vi "GoToControl.vi"(6 "Team":enum16{"Offensive", "Defensive", "Kepper"}(ring), 8 "error in (no error)":errorcluster, 9 "PID Gains Angle":T1={"proportional gain (Kc)"=5.0, "integral time (Ti, min)"=0.0, "derivative time (Td, min)"=-2.0}, 10 "PID Gains XY":T1={"proportional gain (Kc)"=0.005, "integral time (Ti, min)"=0.0, "derivative time (Td, min)"=-0.07}, 11 "Game in":refnum<class "Game.lvclass">) -> (0 "error out":errorcluster, 3 "Game out":refnum<class "Game.lvclass">)   [LabVIEW 2021, in "Game.lvclass"]
uses:
  Game.lvclass
  Game.lvclass/Game.ctl
  Team_class/Team.lvclass/Team.ctl
  Object_class/Object.lvclass/Object.ctl
  Robot_class/Robot.lvclass/Robot.ctl
  Object_class/Read x.vi
  Object_class/Read y.vi
  Robot_class/Read orientation.vi
  Robot_class/Read dest_x.vi
  Robot_class/Read dest_y.vi
  Robot_class/Read dest_orientation.vi
  Robot_class/Read id.vi
  Robot_class/Write v_tang.vi
  Robot_class/Write v_norm.vi
  Robot_class/Write v_ang.vi
  Write OffensiveTeam.vi
  Write DefensiveTeam.vi
  Write KeeperTeam.vi
  Team_class/Read RobotRef.vi
  Team_class/Write RobotRef.vi
  Ally_class/Ally.lvclass
  D:/RoboIme/horie/SSL_AI/Team_class/Team.lvclass
  Robot_class/Robot.lvclass
  D:/RoboIme/horie/SSL_AI/Object_class/Object.lvclass
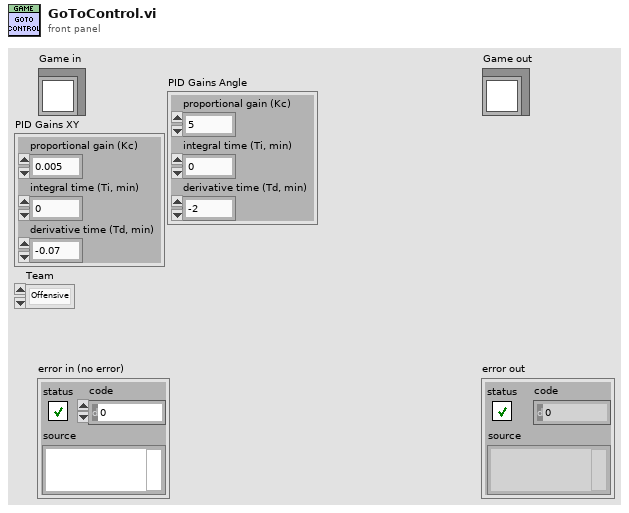
[diagram p1: front panel]
types:
  T1 = cluster{"proportional gain (Kc)":dbl, "integral time (Ti, min)":dbl, "derivative time (Td, min)":dbl}
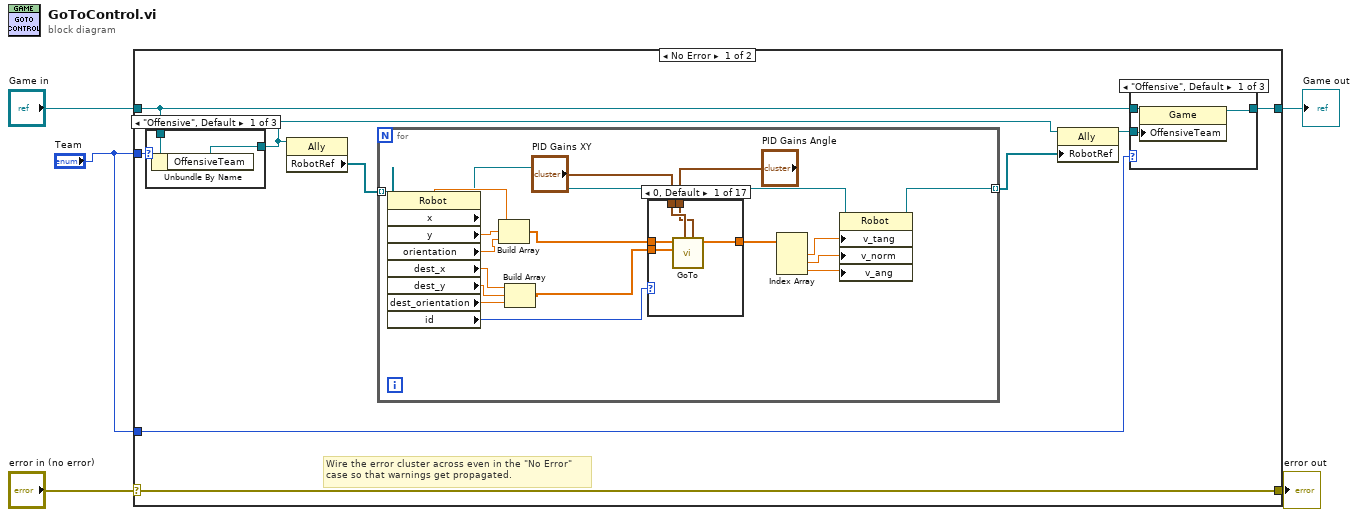
[diagram p0: block diagram]
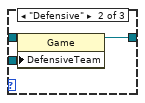
[diagram p2: hidden frame]
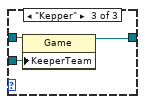
[diagram p3: hidden frame]
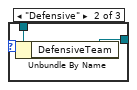
[diagram p4: hidden frame]
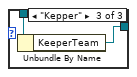
[diagram p5: hidden frame]
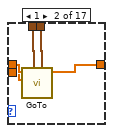
[diagram p6: hidden frame]
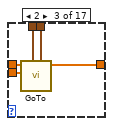
[diagram p7: hidden frame]
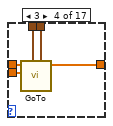
[diagram p8: hidden frame]
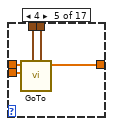
[diagram p9: hidden frame]
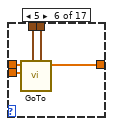
[diagram p10: hidden frame]
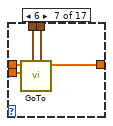
[diagram p11: hidden frame]
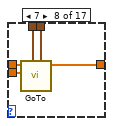
[diagram p12: hidden frame]
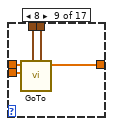
[diagram p13: hidden frame]
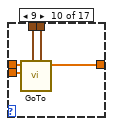
[diagram p14: hidden frame]
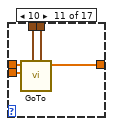
[diagram p15: hidden frame]
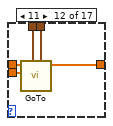
[diagram p16: hidden frame]
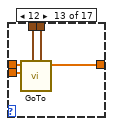
[diagram p17: hidden frame]
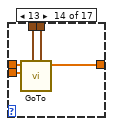
[diagram p18: hidden frame]
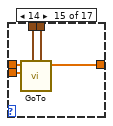
[diagram p19: hidden frame]
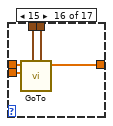
[diagram p20: hidden frame]
diagram:
  n1 = case shown="No Error" "error in (no error)" {
    selector: "error in (no error)" -> [w14 w134]
    tunnel: [w14 w134] -> w4
    tunnel: [w8 w133] -> w2
    tunnel: "Game in" -> [w10 w133]
    tunnel: "Team" -> [w7 _]
    tunnel: "Team" -> [w6 _]
    frame No Error {
      # "Wire the error cluster across even in the \"No Error\"\ncase so that warnings get propagated."
      n2 = case shown="\"Offensive\", Default" w7 {
        tunnel: [w24 w27 w28] -> w12
        tunnel: w10 -> [w25 w26 w29]
        frame "Offensive", Default {
          n3 = Unbundle By Name(w25) -> ("OffensiveTeam"=w24:refnum<class "Ally.lvclass">)
        }
        frame "Defensive" {
          n4 = Unbundle By Name(w26) -> ("DefensiveTeam"=w27:refnum<class "Ally.lvclass">)
        }
        frame "Kepper" {
          n5 = Unbundle By Name(w29) -> ("KeeperTeam"=w28:refnum<class "Ally.lvclass">)
        }
      }
      n6 = property class="Ally"(reference=w12) -> ("RobotRef"=w13:refnum<class "Robot.lvclass">[])  [unwired: 1 in, 2 out]
      n7 = for {
        tunnel: w13 -> [w47] mode=indexing
        tunnel: [w37] -> w11 mode=indexing
        n8 = property class="Robot"(reference=w47) -> (reference out=w42:refnum<class "Robot.lvclass">, "x"=w46:dbl, "y"=w45:dbl, "orientation"=w34:dbl, "dest_x"=w44:dbl, "dest_y"=w43:dbl, "dest_orientation"=w32:dbl, "id"=w30:i32)  [unwired: 1 in, 1 out]
        n9 = Build Array(w46, w45, w34) -> (w33:dbl[])
        n10 = Build Array(w44, w43, w32) -> (w31:dbl[])
        n11 = case shown="0, Default" w30 {
          tunnel: [w50 w57 w62 w67 w72 w77 w82 w87 w92 w97 w102 w107 w112 w117 w122 w127 w132] -> w41
          tunnel: "PID Gains XY" -> [w52 w56 w61 w66 w71 w76 w81 w86 w91 w96 w101 w106 w111 w116 w121 w126 w131]
          tunnel: "PID Gains Angle" -> [w51 w55 w60 w65 w70 w75 w80 w85 w90 w95 w100 w105 w110 w115 w120 w125 w130]
          tunnel: w33 -> [w49 w54 w59 w64 w69 w74 w79 w84 w89 w94 w99 w104 w109 w114 w119 w124 w129]
          tunnel: w31 -> [w48 w53 w58 w63 w68 w73 w78 w83 w88 w93 w98 w103 w108 w113 w118 w123 w128]
          frame 0, Default {
            n12 = call "GoTo.vi"("PID Gains Angle"=w51, "PID Gains XY"=w52, "Target"=w48, "Position"=w49) -> ("Output\nVelocity"=w50:dbl[])  [unwired: 6 in, 1 out]
          }
          frame 1 {
            n13 = call "GoTo.vi"("PID Gains Angle"=w55, "PID Gains XY"=w56, "Target"=w53, "Position"=w54) -> ("Output\nVelocity"=w57:dbl[])  [unwired: 6 in, 1 out]
          }
          frame 2 {
            n14 = call "GoTo.vi"("PID Gains Angle"=w60, "PID Gains XY"=w61, "Target"=w58, "Position"=w59) -> ("Output\nVelocity"=w62:dbl[])  [unwired: 6 in, 1 out]
          }
          frame 3 {
            n15 = call "GoTo.vi"("PID Gains Angle"=w65, "PID Gains XY"=w66, "Target"=w63, "Position"=w64) -> ("Output\nVelocity"=w67:dbl[])  [unwired: 6 in, 1 out]
          }
          frame 4 {
            n16 = call "GoTo.vi"("PID Gains Angle"=w70, "PID Gains XY"=w71, "Target"=w68, "Position"=w69) -> ("Output\nVelocity"=w72:dbl[])  [unwired: 6 in, 1 out]
          }
          frame 5 {
            n17 = call "GoTo.vi"("PID Gains Angle"=w75, "PID Gains XY"=w76, "Target"=w73, "Position"=w74) -> ("Output\nVelocity"=w77:dbl[])  [unwired: 6 in, 1 out]
          }
          frame 6 {
            n18 = call "GoTo.vi"("PID Gains Angle"=w80, "PID Gains XY"=w81, "Target"=w78, "Position"=w79) -> ("Output\nVelocity"=w82:dbl[])  [unwired: 6 in, 1 out]
          }
          frame 7 {
            n19 = call "GoTo.vi"("PID Gains Angle"=w85, "PID Gains XY"=w86, "Target"=w83, "Position"=w84) -> ("Output\nVelocity"=w87:dbl[])  [unwired: 6 in, 1 out]
          }
          frame 8 {
            n20 = call "GoTo.vi"("PID Gains Angle"=w90, "PID Gains XY"=w91, "Target"=w88, "Position"=w89) -> ("Output\nVelocity"=w92:dbl[])  [unwired: 6 in, 1 out]
          }
          frame 9 {
            n21 = call "GoTo.vi"("PID Gains Angle"=w95, "PID Gains XY"=w96, "Target"=w93, "Position"=w94) -> ("Output\nVelocity"=w97:dbl[])  [unwired: 6 in, 1 out]
          }
          frame 10 {
            n22 = call "GoTo.vi"("PID Gains Angle"=w100, "PID Gains XY"=w101, "Target"=w98, "Position"=w99) -> ("Output\nVelocity"=w102:dbl[])  [unwired: 6 in, 1 out]
          }
          frame 11 {
            n23 = call "GoTo.vi"("PID Gains Angle"=w105, "PID Gains XY"=w106, "Target"=w103, "Position"=w104) -> ("Output\nVelocity"=w107:dbl[])  [unwired: 6 in, 1 out]
          }
          frame 12 {
            n24 = call "GoTo.vi"("PID Gains Angle"=w110, "PID Gains XY"=w111, "Target"=w108, "Position"=w109) -> ("Output\nVelocity"=w112:dbl[])  [unwired: 6 in, 1 out]
          }
          frame 13 {
            n25 = call "GoTo.vi"("PID Gains Angle"=w115, "PID Gains XY"=w116, "Target"=w113, "Position"=w114) -> ("Output\nVelocity"=w117:dbl[])  [unwired: 6 in, 1 out]
          }
          frame 14 {
            n26 = call "GoTo.vi"("PID Gains Angle"=w120, "PID Gains XY"=w121, "Target"=w118, "Position"=w119) -> ("Output\nVelocity"=w122:dbl[])  [unwired: 6 in, 1 out]
          }
          frame 15 {
            n27 = call "GoTo.vi"("PID Gains Angle"=w125, "PID Gains XY"=w126, "Target"=w123, "Position"=w124) -> ("Output\nVelocity"=w127:dbl[])  [unwired: 6 in, 1 out]
          }
          frame 16 {
            n28 = call "GoTo.vi"("PID Gains Angle"=w130, "PID Gains XY"=w131, "Target"=w128, "Position"=w129) -> ("Output\nVelocity"=w132:dbl[])  [unwired: 6 in, 1 out]
          }
        }
        n29 = Index Array(array=w41) -> (element #1=w40:dbl, element #2=w39:dbl, element #3=w38:dbl)  [unwired: 3 in]
        n30 = property class="Robot"(reference=w42, "v_tang"=w40, "v_norm"=w39, "v_ang"=w38) -> (reference out=w37:refnum<class "Robot.lvclass">)  [unwired: 1 in, 1 out]
      }
      n31 = property class="Ally"(reference=w12, "RobotRef"=w11) -> (reference out=w9:refnum<class "Ally.lvclass">)  [unwired: 1 in, 1 out]
      n32 = case shown="\"Offensive\", Default" w6 {
        tunnel: w10 -> [w16 w20 w23]
        tunnel: w9 -> [w17 w19 w22]
        tunnel: [w15 w18 w21] -> w8
        frame "Offensive", Default {
          n33 = property class="Game"(reference=w16, "OffensiveTeam"=w17) -> (reference out=w15:refnum<class "Game.lvclass">)  [unwired: 1 in, 1 out]
        }
        frame "Defensive" {
          n34 = property class="Game"(reference=w20, "DefensiveTeam"=w19) -> (reference out=w18:refnum<class "Game.lvclass">)  [unwired: 1 in, 1 out]
        }
        frame "Kepper" {
          n35 = property class="Game"(reference=w23, "KeeperTeam"=w22) -> (reference out=w21:refnum<class "Game.lvclass">)  [unwired: 1 in, 1 out]
        }
      }
    }
    frame Error {
    }
  }
  "error out" <- w4
  "Game out" <- w2
